vi "Example.vi"() -> ()   [LabVIEW 2019, in "MicronTemplateAPIs.lvlib" / "MicronTemplateAPIs.lvclass"]
uses:
  MicronTemplateAPIs.lvclass
  vi.lib/Micron/Base/Client/Typedefs/ServiceDetails.ctl
  9ceadd3c-745e-4cc0-becc-c9896ef65399.vi
  <vilib>/SLL Toolkit/SLL File IO/SLL File IO.lvlib
  vi.lib/Micron/Base/Client/MicronClient.lvclass
panel:
  in  "Connection Type":enum32{"Start New", "Connect Existing"}(tab)
  in  "Mode":string(combo)="Default"
  in  "Path":path
  in  "Port":i32=50051
  in  "ServiceID":string="micron-1"
  in  "UI":string(combo)="show"
  in  "Connection String":string="localhost:50051"
  out "error out":errorcluster
  out "Response":string
  in  "Command":string="Hello Micron!"
  in  "Payload":string="An Open Source Microservice Architecture on top of gRPC from https://github.com/KarthikAbiram/Micron"
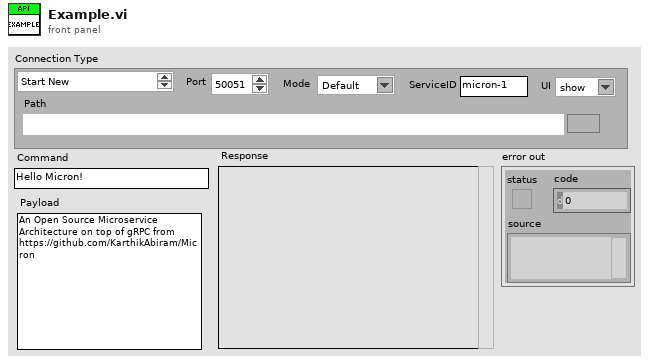
[diagram p1: front panel]
types:
  T1 = typedef "MicronClient.lvclass/ServiceDetails.ctl" = cluster{"MicronPath":path, "Network":string, "ServiceID":string, "Port":i32, "FullyQualifiedName":string, "UI":string, "Args":string, "Mode":string, "AutoRestartOnError?":bool, "Simulate?":bool}
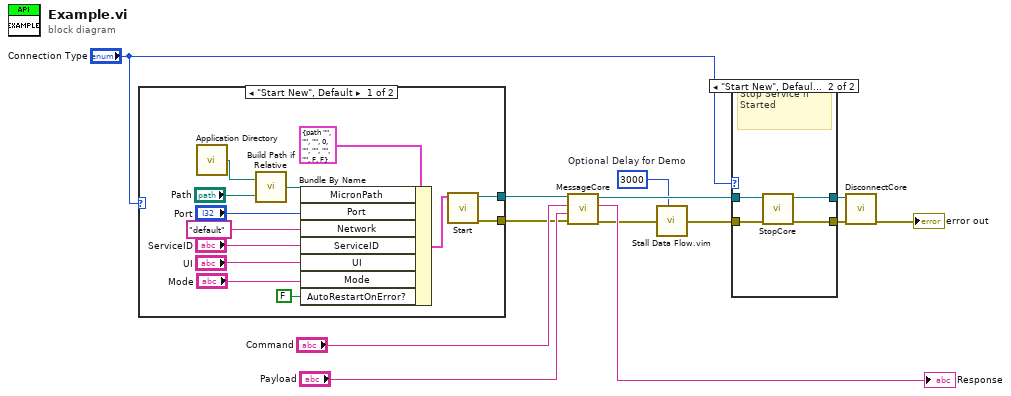
[diagram p0: block diagram]
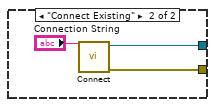
[diagram p3: hidden frame]
diagram:
  w1 = u32 3000  # Optional Delay for Demo
  n1 = case shown="\"Start New\", Default" "Connection Type" {
    tunnel: [w26 w29] -> w9
    tunnel: [w25 w28] -> w8
    frame "Start New", Default {
      n2 = call <vilib>:"Application Directory.vi"() -> ("Application Directory"=w19:path)
      n3 = call <vilib>:"Build Path if Relative.vi"("Relative or Absolute Path"="Path", "Base Path"=w19) -> ("Path Out"=w20:path)
      n4 = Bundle By Name(cluster=T1 {"MicronPath"=path "", "Network"="", "ServiceID"="", "Port"=0, "FullyQualifiedName"="", "UI"="", "Args"="", "Mode"="", "AutoRestartOnError?"=FALSE, "Simulate?"=FALSE} ("Service Details"), "MicronPath"=w20, "Port"="Port", "Network"="default", "ServiceID"="ServiceID", "UI"="UI", "Mode"="Mode", "AutoRestartOnError?"=FALSE) -> (w23:T1)
      n5 = call "Start.vi"("Service Details"=w23) -> ("error out"=w26:errorcluster, "MicronTemplateAPIs out"=w25:refnum<class "MicronTemplateAPIs.lvclass">)  [unwired: 9 in]
    }
    frame "Connect Existing" {
      n6 = call "Connect.vi"("Connection String"="Connection String") -> ("error out"=w29:errorcluster, "MicronTemplateAPIs out"=w28:refnum<class "MicronTemplateAPIs.lvclass">)  [unwired: 9 in]
    }
  }
  n7 = call-dynamic "MessageCore.vi"("error in (no error)"=w9, "Payload"="Payload", "Command"="Command", "GRPCClient in"=w8) -> ("error out"=w7:errorcluster, "Response"=→"Response":string, "GRPCClient out"=w6:refnum<class "MicronTemplateAPIs.lvclass">)  [unwired: 5 in]
  n8 = call "Stall Data Flow.vim"("value in"=w7, "milliseconds to wait"=w1) -> ("value out"=w2:errorcluster)  [unwired: 1 out]
  n9 = case shown="\"Start New\", Default" "Connection Type" {
    tunnel: w2 -> [w31 w35]
    tunnel: w6 -> [w30 w34]
    tunnel: [w30 w33] -> w5
    tunnel: [w31 w32] -> w4
    frame "Connect Existing" {
    }
    frame "Start New", Default {
      # "Stop Service if Started"
      n10 = call-dynamic "StopCore.vi"("error in (no error)"=w35, "MicronGRPCClient in"=w34) -> ("error out"=w32:errorcluster, "MicronGRPCClient out"=w33:refnum<class "MicronTemplateAPIs.lvclass">)  [unwired: 7 in, 1 out]
    }
  }
  n11 = call-dynamic "DisconnectCore.vi"("error in (no error)"=w4, "GRPCClient in"=w5) -> ("error out"=→"error out":errorcluster)  [unwired: 8 in, 1 out]
